vi "HandleError.vi"(8 "error in (no error)":errorcluster, 9 "Causing VI":string, 10 "Calling VI":string) -> (0 "error out":errorcluster)   [LabVIEW 2013]
uses:
  <vilib>/Rock Robotics/Network Tables/SD Write Numeric Array.vi
  <vilib>/Rock Robotics/Network Tables/SD Write Boolean Array.vi
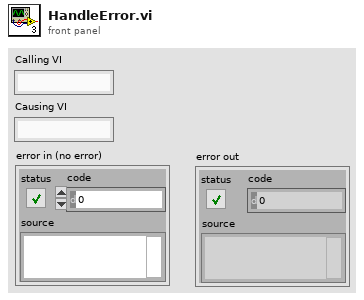
[diagram p1: front panel]
types:
  T1 = cluster{"Boolean":bool, "Numeric":i32, "String":string}
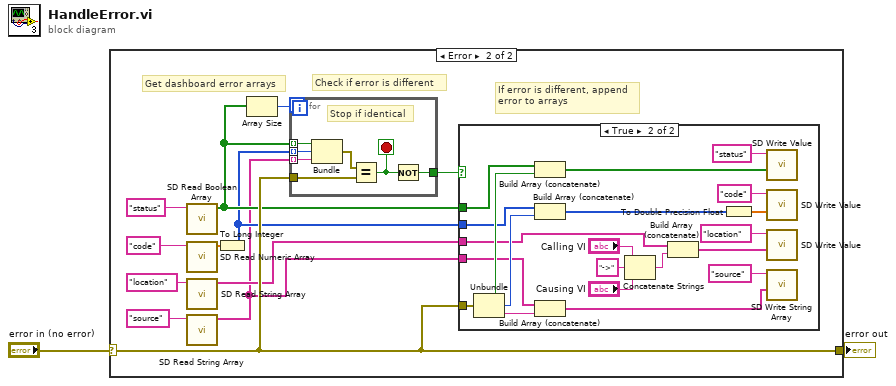
[diagram p0: block diagram]
diagram:
  n1 = case shown="Error" "error in (no error)" {
    selector: "error in (no error)" -> [w3 w10]
    tunnel: [w3 w10] -> w1
    frame No Error {
    }
    frame Error {
      # "Check if error is different"
      # "If error is different, append\nerror to arrays"
      # "Get dashboard error arrays"
      n2 = call <vilib>:"SD Read Boolean Array.vi"("Name"="status") -> ("Boolean Array"=w8:bool[])  [unwired: 8 in, 2 out]
      n3 = call <vilib>:"SD Read Numeric Array.vi"("Name"="code") -> ("Numeric Array"=w12:dbl[])  [unwired: 8 in, 2 out]
      n4 = call <vilib>:"SD Read String Array.vi"("Name"="location") -> ("String Array"=w5:string[])  [unwired: 9 in, 1 out]
      n5 = call <vilib>:"SD Read String Array.vi"("Name"="source") -> ("String Array"=w4:string[])  [unwired: 9 in, 1 out]
      n6 = To Long Integer(number=w12) -> (32bit integer=w7:i32[])
      n7 = Array Size(array=w8) -> (size(s)=w11:i32)
      n8 = for {
        N: w11 -> [_]
        tunnel: w10 -> [w40]
        tunnel: w8 -> [w43] mode=indexing
        tunnel: w7 -> [w42] mode=indexing
        tunnel: w4 -> [w41] mode=indexing
        tunnel: [w37] -> w9
        stop <- w38 stop-if-true
        # "Stop if identical"
        n9 = Bundle("Boolean"=w43, "Numeric"=w42, "String"=w41) -> (w39:T1)  [unwired: 1 in]
        n10 = Equal?(x=w39, y=w40) -> (x = y?=w38:bool)
        n11 = Not(x=w38) -> (.not. x?=w37:bool)
      }
      n12 = case shown="True" w9 {
        tunnel: w10 -> [_ w36]
        tunnel: w8 -> [_ w29]
        tunnel: w7 -> [_ w26]
        tunnel: w5 -> [_ w19]
        tunnel: w4 -> [_ w20]
        frame False {
        }
        frame True {
          n13 = Unbundle(w36) -> ("status"=w28:bool, "code"=w25:i32, "source"=w21:string)
          n14 = Build Array (concatenate)(w29, w28) -> (w27:bool[])
          n15 = Build Array (concatenate)(w26, w25) -> (w24:i32[])
          n16 = Build Array (concatenate)(w20, w21) -> (w17:string[])
          n17 = Concatenate Strings("Calling VI", "->" ("string"), "Causing VI") -> (w18:string)
          n18 = Build Array (concatenate)(w19, w18) -> (w16:string[])
          n19 = To Double Precision Float(number=w24) -> (double precision float=w23:dbl[])
          n20 = call-poly <vilib>:"SD Write Value.vi"("Boolean Array"=w27, "Name"="status") -> ()  [unwired: 8 in, 2 out]
          n21 = call-poly <vilib>:"SD Write Value.vi"("Numeric Array"=w23, "Name"="code") -> ()  [unwired: 8 in, 2 out]
          n22 = call-poly <vilib>:"SD Write Value.vi"("String Array"=w16, "Name"="location") -> ()  [unwired: 8 in, 2 out]
          n23 = call <vilib>:"SD Write String Array.vi"("String Array"=w17, "Name"="source") -> ()  [unwired: 8 in, 2 out]
        }
      }
    }
  }
  "error out" <- w1
